vi "浊度电极校准.vi"() -> ()   [LabVIEW 2016, in "斯坦道多参数.lvlib"]
uses:
  <vilib>/Utility/miscctls.llb/LVPointTypeDef.ctl
  <vilib>/Utility/miscctls.llb/LVPositionTypeDef.ctl
  <vilib>/Analysis/NI_AALBase.lvlib
panel:
  out "通讯状态":string
  out "电极状态标志":u16(ring) items=["OK"=0, "第一点校正通过"=1, "第二点校正通过"=2, "悬浮物两点校准第一点校正通过"=11, "悬浮物两点校准第二点校正通过"=12, "浊度三点校正第一点校正通过"=31, "浊度三点校正第二点校正通过"=32, "浊度三点校正第三点校正通过"=33]
  out "第三点校准值":dbl
  out "标液3":dbl
  out "第二点校准值":dbl
  out "第一点校准值":dbl
  in  "校准停止":bool
  in  "校准启动":bool
  in  "校准模式":enum16{"两点校准", "单点校准", "三点校准"}(ring)
  out "最小值":sgl format="%#.2f"
  out "最大值":sgl format="%#.2f"
  out "波形图表":sgl(graph) caption="历史曲线"
  out "mean":dbl caption="均值" format="%#.2f"
  out "standard deviation":dbl caption="标准差" format="%#.2f"
  out "变异系数":dbl format="%#.6f"
  out "测量值":dbl
  out "提示":string
  out "标液2":dbl
  out "标液1":dbl
  out "原始读取值":dbl caption="信号值"
  out "偏移值补偿":dbl
  out "电极斜率":dbl
  out "电极零点":dbl
  # "浊度电极设定"
  # "NTU"
  # "%"
  # "NTU"
  # "NTU"
  # "NTU"
  # "请选择校准模式:"
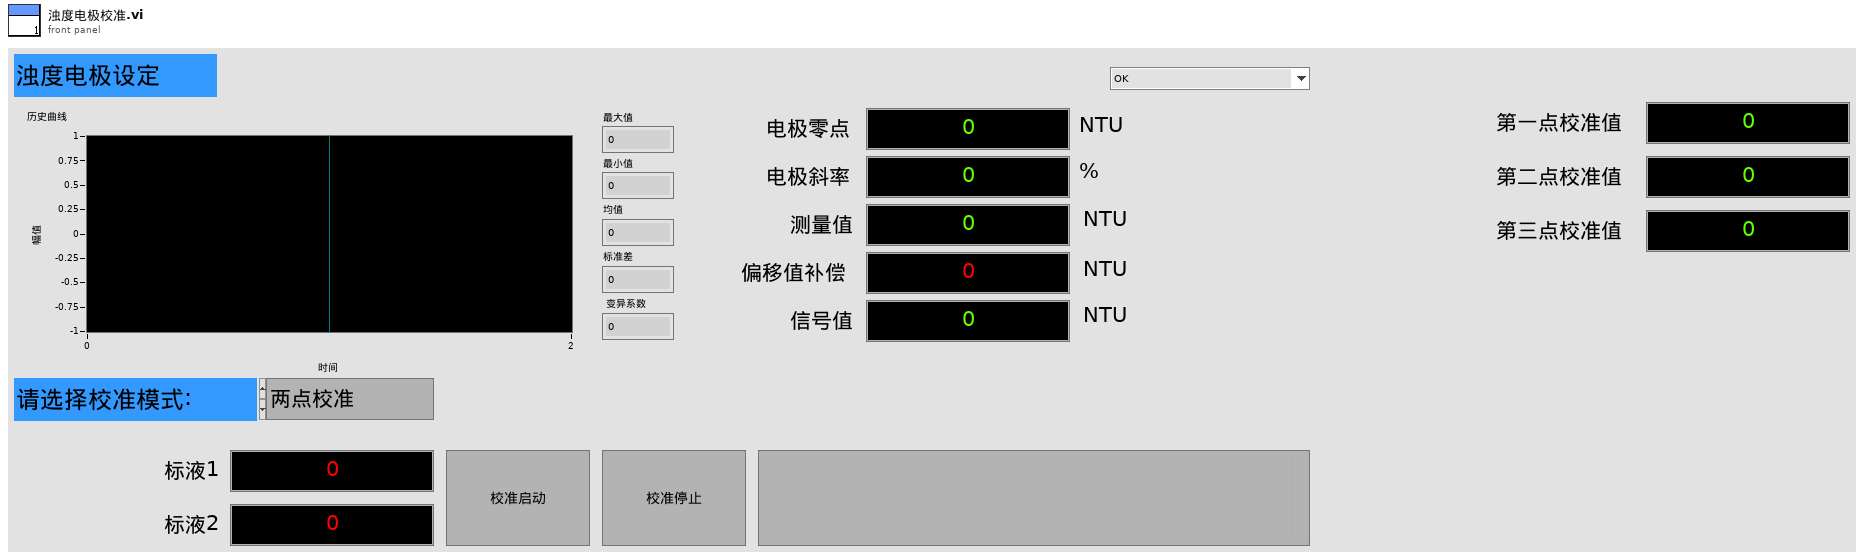
[diagram p1: front panel]
types:
  T1 = typedef "LVPointTypeDef.ctl" = cluster{"Horizontal":i16, "Vertical":i16}
  T2 = typedef "斯坦道多参数.lvlib/校准步骤.ctl" = enum16{"待机", "放置第一点标液", "第一点校准启动", "第一点校准写入", "第一点校准失败", "放置第二点标液", "第二点校准启动", "第二点校准写入", "第二点校准失败", "放置第三点标液", "第三点校准启动", "第三点校准写入", "第三点校准失败", "校准结果写入", "校准结束"}
  T3 = cluster{"电极状态标志":u16, "电极型号标志":u16, "浊度测量值":sgl, "温度测量值":sgl, "浊度信号值":sgl, "浊度偏移修正值":sgl, "温度偏移修正值":sgl, "手动温度补偿值":sgl, "浊度电极零点":sgl, "浊度电极斜率":sgl, "第1点标准值记录":sgl, "第1点信号值记录":sgl, "第1点温度值记录":sgl, "第2点标准值记录":sgl, "第2点信号值记录":sgl, "第2点温度值记录":sgl, "命令滤波设定":u16, "温度模式":enum16{"ATC", "MTC"}, "生产批次":u16, "电极序号":u16, "串口地址":u16, "串口波特率":enum16{"9600", "19200", "115200"}, "串口校验位":enum16{"NONE", "ODD", "EVEN"}, "串口停止位":enum16{"1bit", "2bit"}, "第一点标准值":sgl, "第二点标准值":sgl, "第三点标准值":sgl}
  T4 = typedef "LVPositionTypeDef.ctl" = cluster{"Left":i32, "Top":i32}
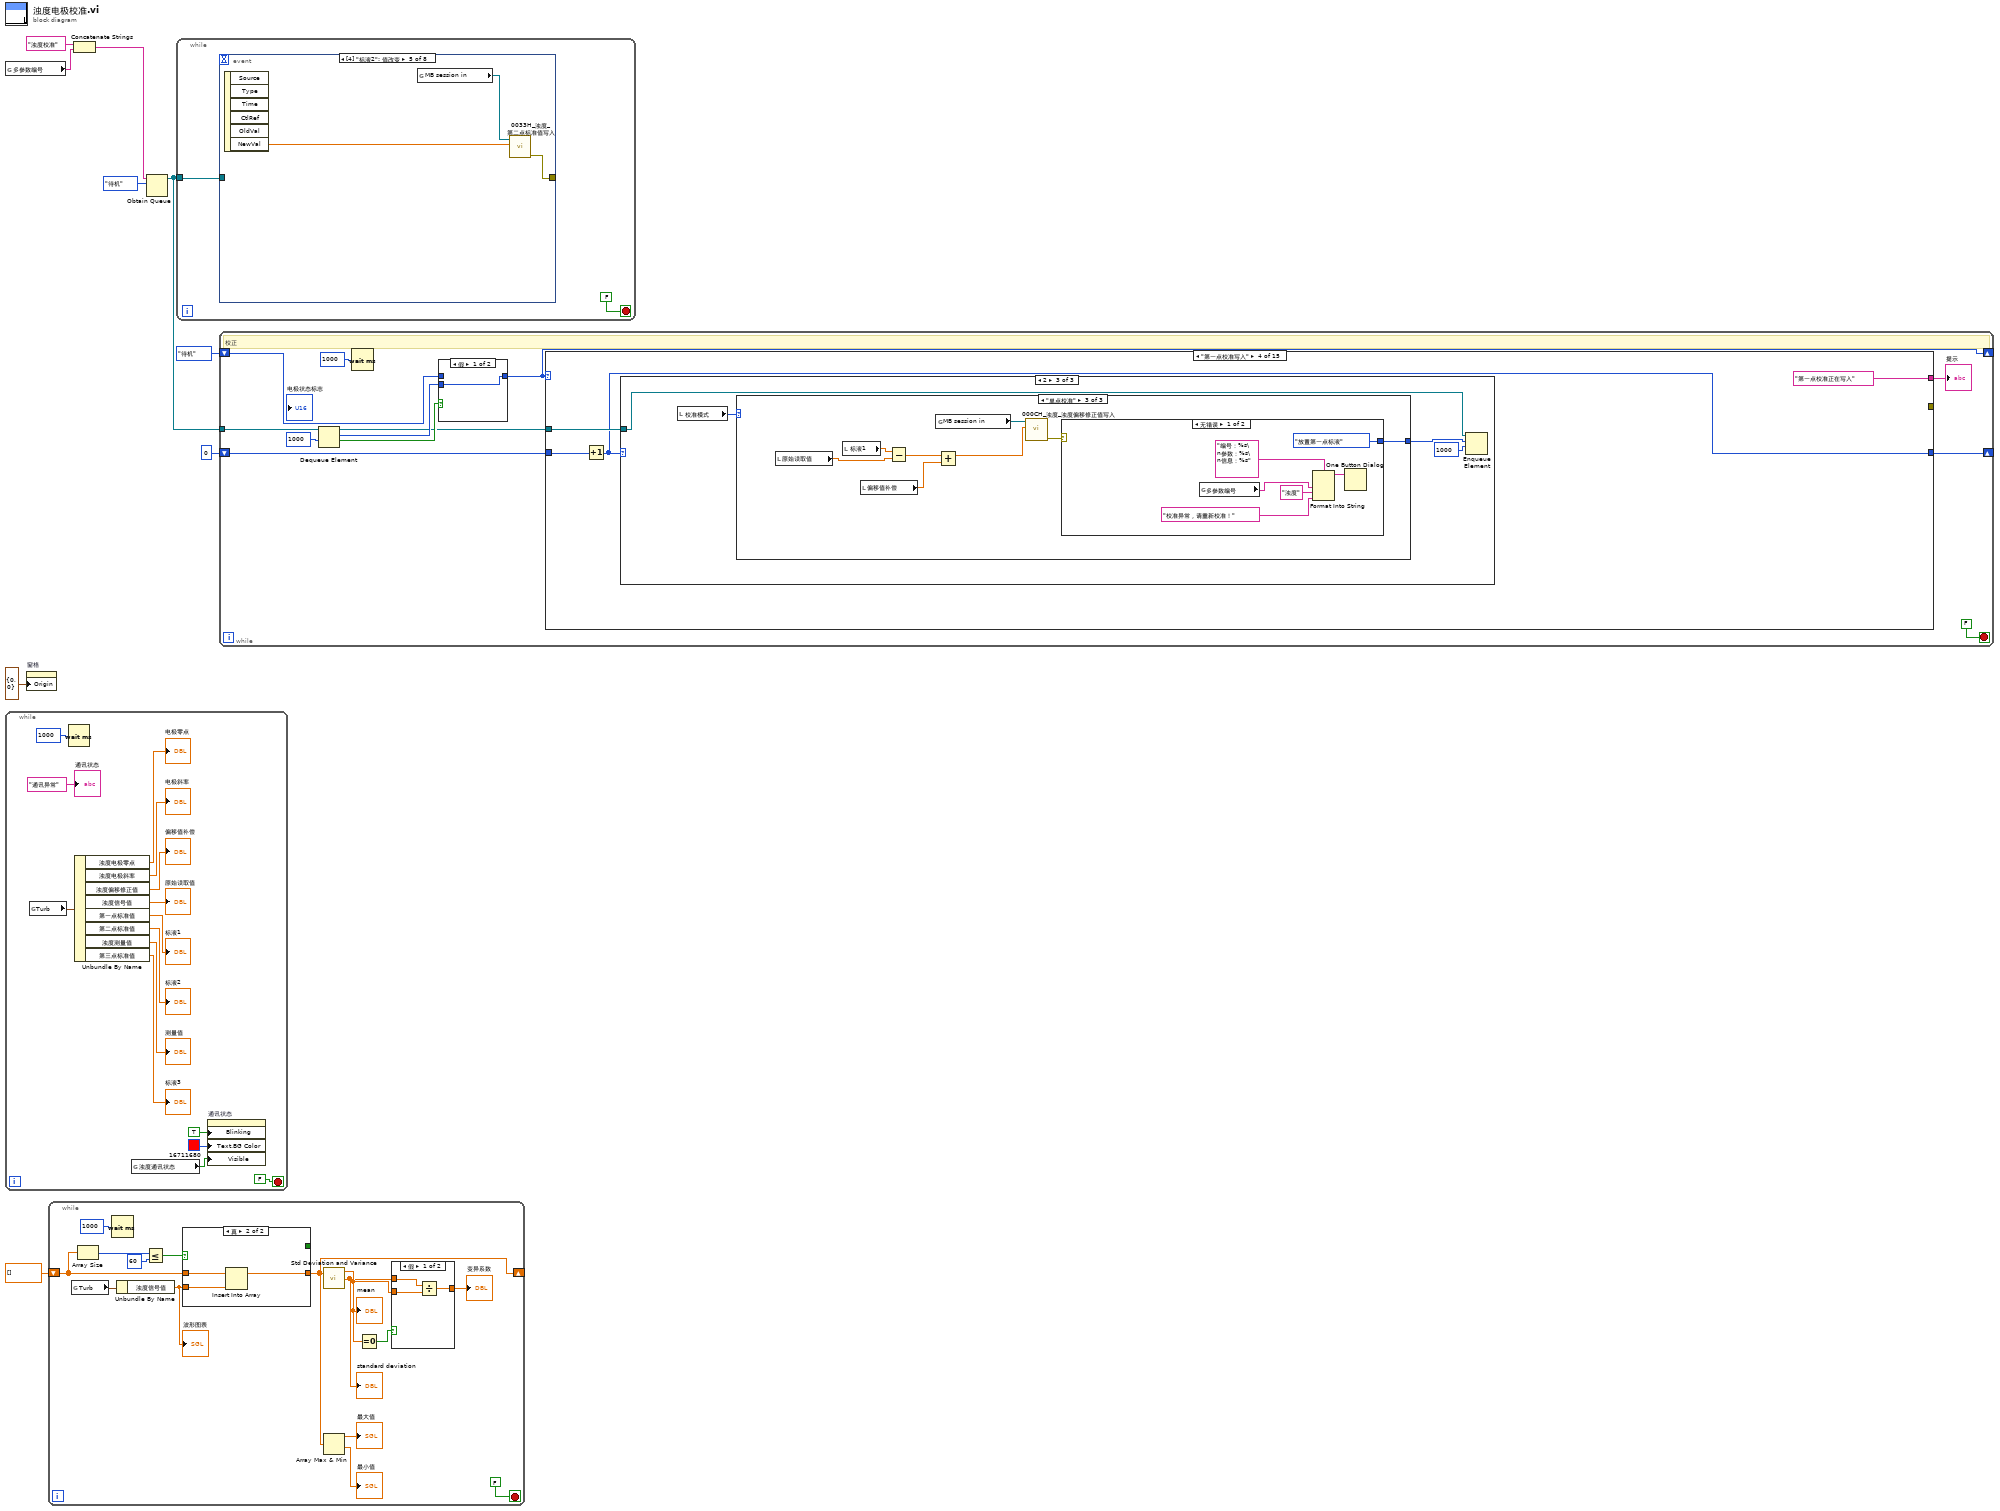
[diagram p0: block diagram]
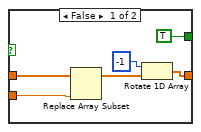
[diagram p3: hidden frame]
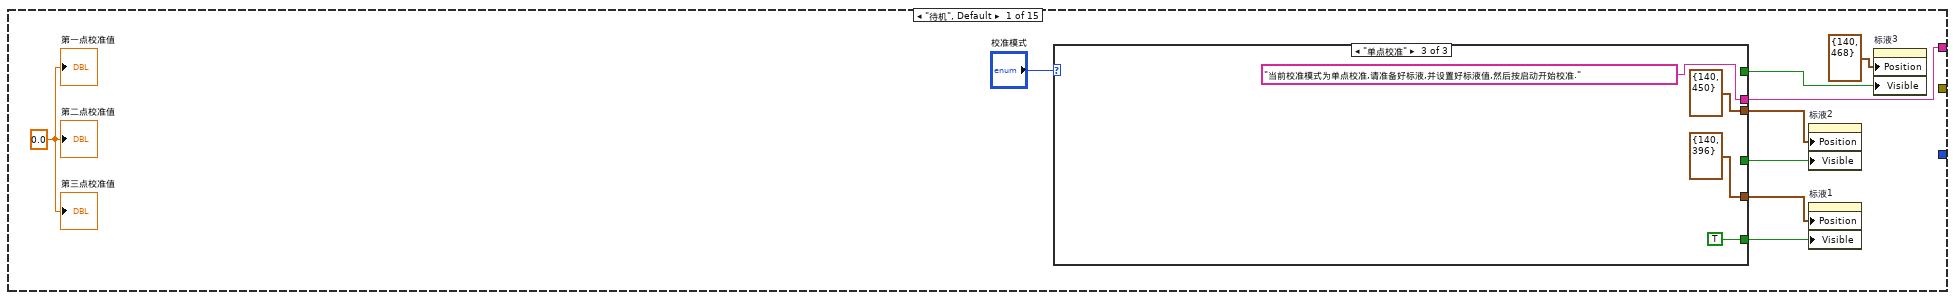
[diagram p5: hidden frame]
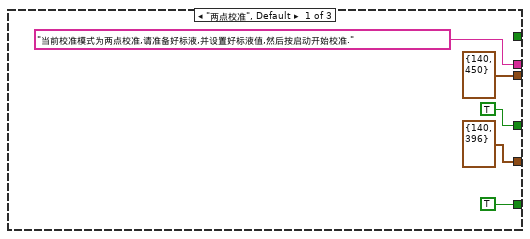
[diagram p6: hidden frame]
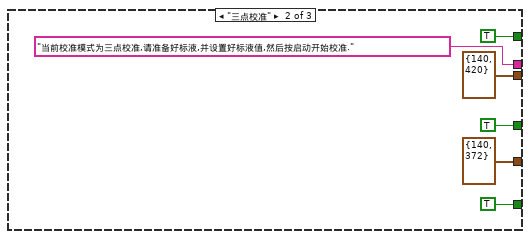
[diagram p7: hidden frame]
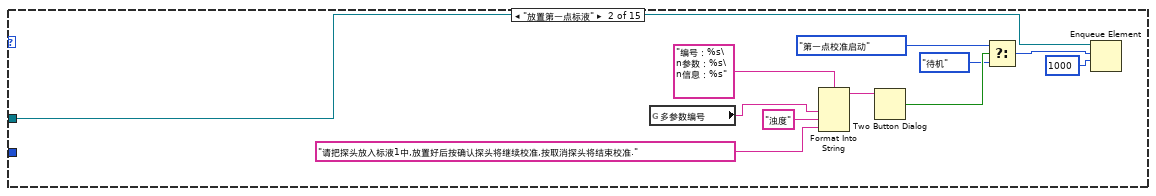
[diagram p8: hidden frame]
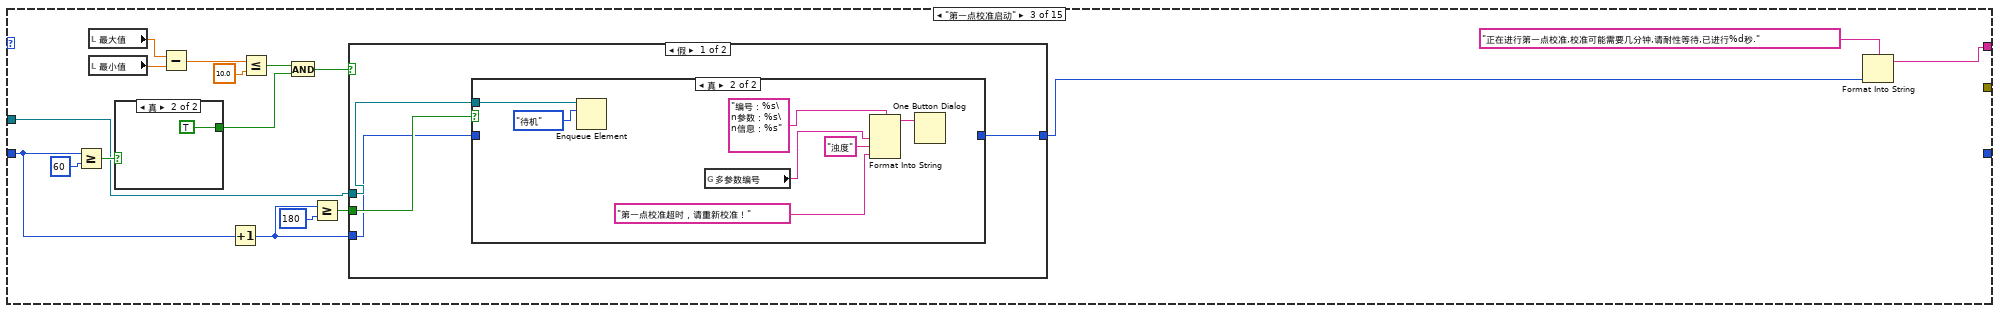
[diagram p9: hidden frame]
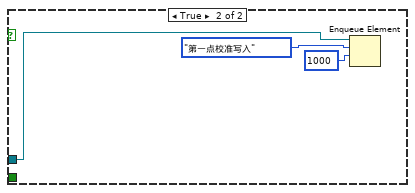
[diagram p11: hidden frame]
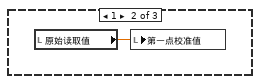
[diagram p14: hidden frame]
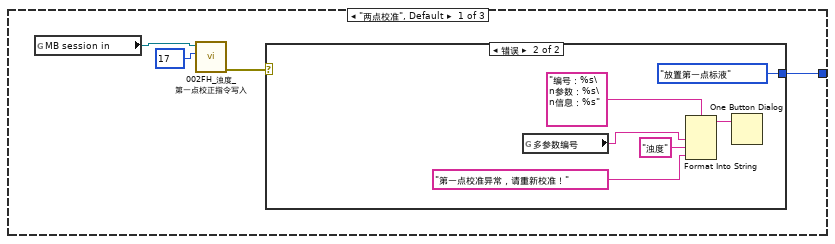
[diagram p15: hidden frame]
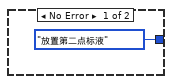
[diagram p16: hidden frame]
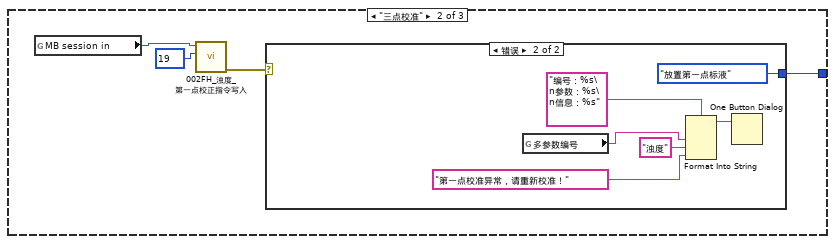
[diagram p17: hidden frame]
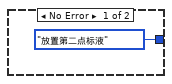
[diagram p18: hidden frame]
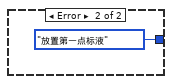
[diagram p19: hidden frame]
diagram:
  n1 = global read "多参数全局变量.vi" "多参数编号"() -> (w1:string)
  n2 = while {
    stop <- FALSE stop-if-true
    n3 = global read "国弘过程全局变量.vi" "Turb"() -> (w22:T3)
    n4 = Wait (ms)(milliseconds to wait=u32 1000 ("等待时间（毫秒）")) -> ()  [unwired: 1 out]
    n5 = Unbundle By Name(w22) -> ("浊度电极零点"=→"电极零点":sgl, "浊度电极斜率"=→"电极斜率":sgl, "浊度偏移修正值"=→"偏移值补偿":sgl, "浊度信号值"=→"原始读取值":sgl, "第一点标准值"=→"标液1":sgl, "第二点标准值"=→"标液2":sgl, "浊度测量值"=→"测量值":sgl, "第三点标准值"=→"标液3":sgl)
    n6 = global read "多参数全局变量.vi" "浊度通讯状态"() -> (w10:bool)
    n7 = property on="通讯状态" class="Str"("Blinking"=TRUE ("闪烁"), "Text.BG Color"=u32 16711680, "Visible"=w10) -> ()  [unwired: 2 in, 2 out]
    "通讯状态" <- "通讯异常" ("当前串口")
  }
  n8 = property on="窗格" class="Pane"("Origin"=T1 {"Horizontal"=0, "Vertical"=0} ("原点")) -> ()  [unwired: 2 in, 2 out]
  n9 = while {
    shift-right: [w28] -> _
    shift-left: sgl[] [] -> [w35]
    stop <- FALSE stop-if-true
    n10 = global read "国弘过程全局变量.vi" "Turb"() -> (w29:T3)
    n11 = Array Size(array=w35) -> (size(s)=w37:i32)
    n12 = Wait (ms)(milliseconds to wait=u32 1000 ("等待时间（毫秒）")) -> ()  [unwired: 1 out]
    n13 = Unbundle By Name(w29) -> ("浊度信号值"=w25:sgl)
    "波形图表" <- w25
    n14 = Less Or Equal?(x=w37, y=60) -> (x <= y?=w36:bool)
    n15 = case shown="真" w36 {
      tunnel: w35 -> [w48 w51]
      tunnel: w25 -> [w46 w50]
      tunnel: [w44 w49] -> w28
      tunnel: [TRUE _] -> _
      frame False {
        n16 = Replace Array Subset(array=w48, new element=w46) -> (w47:sgl[])  [unwired: 1 in]
        n17 = Rotate 1D Array(1:w47, 2:-1 ("n")) -> (0:w44:sgl[])
      }
      frame True {
        n18 = Insert Into Array(array=w51, new element=w50) -> (w49:sgl[])  [unwired: 1 in]
      }
    }
    n19 = call <vilib>:"Std Deviation and Variance.vi"("X"=w28) -> ("mean"=w33:dbl, "standard deviation"=w32:dbl)  [unwired: 1 in, 1 out]
    "mean" <- w33
    "standard deviation" <- w32
    n20 = Array Max & Min(array=w28) -> (max value=→"最大值":sgl, min value=→"最小值":sgl)  [unwired: 2 out]
    n21 = Equal To 0?(x=w33) -> (x = 0?=w34:bool)
    n22 = case shown="假" w34 {
      tunnel: w32 -> [w42 _]
      tunnel: [w41 _] -> w31
      tunnel: w33 -> [w40 _]
      frame False {
        n23 = Divide(x=w42, y=w40) -> (x/y=w41:dbl)
      }
      frame True {
      }
    }
    "变异系数" <- w31
  }
  n24 = Concatenate Strings("浊度校准" ("名称（未命名）"), w1) -> (w2:string)
  n25 = Obtain Queue(name (unnamed)=w2, element data type=校准步骤."待机" ("枚举")) -> (queue out=w4:refnum<queue>)  [unwired: 3 in, 2 out]
  n26 = while {
    tunnel: w4 -> [w52]
    stop <- FALSE stop-if-true
    n27 = event shown="[4] \"标液2\": 值改变" {
      selector: _ -> [_ _ _ _ _ _ _ _]
      dyn-events: _ -> [_ _ _ _ _ _ _ _]
      timeout: _ -> [_ _ _ _ _ _ _ _]
      tunnel: [_ _ w59 w62 w66 w69 _ _] -> _
      tunnel: w52 -> [_ _ _ _ _ _ w70 w72]
      event Timeout {
        n28 = event-data() -> ()  [unwired: 1 in, 3 out]
      }
      event "偏移值补偿", "标液1", "标液2", "标液3": Mouse Down {
        n29 = event-data() -> ("CtlRef"=w54:refnum<vi>)  [unwired: 1 in, 7 out]
        n30 = property class="DigNum (严格)"(reference=w54) -> (reference out=w55:refnum<vi>, "Value"=w56:dbl)  [unwired: 1 in, 1 out]
        n31 = call "数字键盘.vi"("OldNumber"=w56) -> ("NewNumber"=w57:dbl)  [unwired: 1 in]
        n32 = property class="DigNum (严格)"(reference=w55, "Val(Sgnl)"=w57) -> ()  [unwired: 1 in, 2 out]
      }
      event "偏移值补偿": Value Change {
        n33 = event-data() -> ("NewVal"=w60:dbl)  [unwired: 1 in, 5 out]
        n34 = global read "多参数全局变量.vi" "MB session in"() -> (w58:refnum<class "MB_Master.lvclass">)
        n35 = call "000CH_浊度_浊度偏移修正值写入.vi"("数值"=w60, "MB session in"=w58) -> ("error out"=w59:errorcluster)  [unwired: 8 in, 1 out]
      }
      event "标液1": Value Change {
        n36 = event-data() -> ("NewVal"=w63:dbl)  [unwired: 1 in, 5 out]
        n37 = global read "多参数全局变量.vi" "MB session in"() -> (w61:refnum<class "MB_Master.lvclass">)
        n38 = call "0030H_浊度_第一点标准值写入.vi"("数值"=w63, "MB session in"=w61) -> ("error out"=w62:errorcluster)  [unwired: 8 in, 1 out]
      }
      event "标液2": Value Change {
        n39 = event-data() -> ("NewVal"=w65:dbl)  [unwired: 1 in, 5 out]
        n40 = global read "多参数全局变量.vi" "MB session in"() -> (w64:refnum<class "MB_Master.lvclass">)
        n41 = call "0033H_浊度_第二点标准值写入.vi"("数值"=w65, "MB session in"=w64) -> ("error out"=w66:errorcluster)  [unwired: 8 in, 1 out]
      }
      event "标液3": Value Change {
        n42 = event-data() -> ("NewVal"=w68:dbl)  [unwired: 1 in, 5 out]
        n43 = global read "多参数全局变量.vi" "MB session in"() -> (w67:refnum<class "MB_Master.lvclass">)
        n44 = call "0036H_浊度_第三点标准值写入.vi"("数值"=w68, "MB session in"=w67) -> ("error out"=w69:errorcluster)  [unwired: 8 in, 1 out]
      }
      event "校准启动": Value Change {
        n45 = event-data() -> ()  [unwired: 1 in, 6 out]
        n46 = Enqueue Element(queue=w70, element=校准步骤."放置第一点标液" ("元素")) -> ()  [unwired: 2 in, 3 out]
      }
      event "校准停止": Value Change {
        n47 = event-data() -> ()  [unwired: 1 in, 6 out]
        n48 = Flush Queue(queue=w72) -> (queue out=w73:refnum<queue>)  [unwired: 1 in, 2 out]
        n49 = Enqueue Element(queue=w73, element=校准步骤."待机" ("元素"), timeout in ms (-1)=1000 ("超时毫秒(-1)")) -> ()  [unwired: 1 in, 3 out]
      }
    }
  }
  n50 = while "While循环" {
    shift-right: [w77] -> _
    shift-left: 校准步骤."待机" ("枚举") -> [w79]
    shift-right: [w76] -> _
    shift-left: 0 -> [w85]
    tunnel: w4 -> [w80]
    stop <- FALSE stop-if-true
    # "校正"
    n51 = Dequeue Element(queue=w80, timeout in ms (-1)=1000 ("超时毫秒(-1)")) -> (queue out=w78:refnum<queue>, element=w81:T2, timed out?=w82:bool)  [unwired: 1 in, 1 out]
    n52 = Wait (ms)(milliseconds to wait=u32 1000 ("等待时间（毫秒）")) -> ()  [unwired: 1 out]
    n53 = case shown="假" w82 {
      tunnel: w81 -> [w88 _]
      tunnel: [w88 w89] -> w77
      tunnel: w79 -> [_ w89]
      frame False {
      }
      frame True {
      }
    }
    n54 = case shown="\"第一点校准写入\"" w77 {
      tunnel: [w97 _ w125 "第一点校准正在写入" ("提示") _ _ w217 "第二点校准正在写入" ("提示") "第二点校准失败" ("提示") _ "第三点校准正在写入" ("提示") w313 "第三点校准失败" ("提示") w347 w386] -> w84
      tunnel: w85 -> [_ _ w127 w160 _ _ w218 w250 _ _ w295 w314 _ _ _]
      tunnel: [_ _ _ w158 _ _ w216 w248 _ _ w293 w312 _ _ _] -> w76
      tunnel: w78 -> [_ w119 w128 w159 _ w209 w219 w249 _ w287 w294 w315 _ w354 _]
      tunnel: [_ _ _ _ _ _ _ _ _ _ _ _ _ w352 _] -> _
      frame "待机", Default {
        w90 = 0.0 ("第一点校准值")
        n55 = case shown="\"单点校准\"" "校准模式" {
          tunnel: ["当前校准模式为两点校准,请准备好标液,并设置好标液值,然后按启动开始校准." ("提示") "当前校准模式为三点校准,请准备好标液,并设置好标液值,然后按启动开始校准." ("提示") "当前校准模式为单点校准,请准备好标液,并设置好标液值,然后按启动开始校准." ("提示")] -> w97
          tunnel: [TRUE ("可见") TRUE ("可见") _] -> w93
          tunnel: [T4 {"Left"=140, "Top"=396} ("位置") T4 {"Left"=140, "Top"=372} ("位置") T4 {"Left"=140, "Top"=396} ("位置")] -> w96
          tunnel: [T4 {"Left"=140, "Top"=450} ("位置 2") T4 {"Left"=140, "Top"=420} ("位置 2") T4 {"Left"=140, "Top"=450} ("位置 2")] -> w95
          tunnel: [_ TRUE ("可见") _] -> w92
          tunnel: [TRUE ("可见") TRUE ("可见") TRUE ("可见")] -> w91
          frame "两点校准", Default {
          }
          frame "三点校准" {
          }
          frame "单点校准" {
          }
        }
        n56 = property on="标液2" class="DigNum (严格)"("Position"=w95, "Visible"=w93) -> ()  [unwired: 2 in, 2 out]
        n57 = property on="标液1" class="DigNum (严格)"("Position"=w96, "Visible"=w91) -> ()  [unwired: 2 in, 2 out]
        n58 = property on="标液3" class="DigNum (严格)"("Position"=T4 {"Left"=140, "Top"=468} ("位置 3"), "Visible"=w92) -> ()  [unwired: 2 in, 2 out]
        "第一点校准值" <- w90
        "第二点校准值" <- w90
        "第三点校准值" <- w90
      }
      frame "放置第一点标液" {
        n59 = global read "多参数全局变量.vi" "多参数编号"() -> (w117:string)
        n60 = Format Into String(format string="编号：%s\n参数：%s\n信息：%s" ("格式字符串"), w117, "浊度" ("输入 2"), "请把探头放入标液1中,放置好后按确认探头将继续校准,按取消探头将结束校准." ("消息")) -> (resulting string=w114:string)  [unwired: 2 in, 1 out]
        n61 = Two Button Dialog(message=w114) -> (T button?=w123:bool)  [unwired: 2 in]
        n62 = Select(t=校准步骤."第一点校准启动" ("元素"), s=w123, f=校准步骤."待机" ("元素")) -> (s? t:f=w120:T2)
        n63 = Enqueue Element(queue=w119, element=w120, timeout in ms (-1)=1000 ("超时毫秒(-1)")) -> ()  [unwired: 1 in, 3 out]
      }
      frame "第一点校准启动" {
        n64 = Greater Or Equal?(x=w127, y=60) -> (x >= y?=w134:bool)
        n65 = local read "最大值"() -> (w137:sgl)
        n66 = local read "最小值"() -> (w136:sgl)
        n67 = case shown="真" w134 {
          tunnel: [_ TRUE] -> w135
          frame False {
          }
          frame True {
          }
        }
        n68 = Subtract(x=w137, y=w136) -> (x-y=w138:sgl)
        n69 = Increment(x=w127) -> (x+1=w141:i32)
        n70 = Less Or Equal?(x=w138, y=10.0) -> (x <= y?=w131:bool)
        n71 = And(x=w131, y=w135) -> (x .and. y?=w139:bool)
        n72 = Greater Or Equal?(x=w141, y=180) -> (x >= y?=w140:bool)
        n73 = case shown="假" w139 {
          tunnel: w128 -> [w144 w156]
          tunnel: w140 -> [w145 _]
          tunnel: w141 -> [w143 _]
          tunnel: [w142 _] -> w126
          frame False {
            n74 = case shown="真" w145 {
              tunnel: w144 -> [_ w153]
              tunnel: w143 -> [w146 _]
              tunnel: [w146 _] -> w142
              frame False {
              }
              frame True {
                n75 = Enqueue Element(queue=w153, element=校准步骤."待机" ("元素")) -> ()  [unwired: 2 in, 3 out]
                n76 = global read "多参数全局变量.vi" "多参数编号"() -> (w150:string)
                n77 = Format Into String(format string="编号：%s\n参数：%s\n信息：%s" ("格式字符串"), w150, "浊度" ("输入 2"), "第一点校准超时，请重新校准！" ("error source (\" \")")) -> (resulting string=w148:string)  [unwired: 2 in, 1 out]
                n78 = One Button Dialog(message=w148) -> ()  [unwired: 1 in, 1 out]
              }
            }
          }
          frame True {
            n79 = Enqueue Element(queue=w156, element=校准步骤."第一点校准写入" ("元素"), timeout in ms (-1)=1000 ("超时毫秒(-1)")) -> ()  [unwired: 1 in, 3 out]
          }
        }
        n80 = Format Into String(format string="正在进行第一点校准,校准可能需要几分钟,请耐性等待,已进行%d秒." ("格式字符串"), w126) -> (resulting string=w125:string)  [unwired: 2 in, 1 out]
      }
      frame "第一点校准写入" {
        n81 = Increment(x=w160) -> (x+1=w158:i32)
        n82 = case shown="2" w158 {
          tunnel: w159 -> [_ _ w166]
          frame 0, Default {
          }
          frame 1 {
            n83 = local read "原始读取值"() -> (w162:dbl)
            n84 = local write "第一点校准值"(w162) -> ()
          }
          frame 2 {
            n85 = local read "校准模式"() -> (w165:enum16{"两点校准", "单点校准", "三点校准"})
            n86 = case shown="\"单点校准\"" w165 {
              tunnel: [w167 w178 w191] -> w164
              frame "两点校准", Default {
                n87 = global read "多参数全局变量.vi" "MB session in"() -> (w170:refnum<class "MB_Master.lvclass">)
                n88 = call "002FH_浊度_第一点校正指令写入.vi"("数值"=u16 17, "MB session in"=w170) -> ("error out"=w168:errorcluster)  [unwired: 8 in, 1 out]
                n89 = case shown="错误" w168 {
                  tunnel: [校准步骤."放置第二点标液" ("元素") 校准步骤."放置第一点标液" ("元素")] -> w167
                  frame No Error {
                  }
                  frame Error {
                    n90 = global read "多参数全局变量.vi" "多参数编号"() -> (w176:string)
                    n91 = Format Into String(format string="编号：%s\n参数：%s\n信息：%s" ("格式字符串"), w176, "浊度" ("输入 2"), "第一点校准异常，请重新校准！" ("error source (\" \")")) -> (resulting string=w175:string)  [unwired: 2 in, 1 out]
                    n92 = One Button Dialog(message=w175) -> ()  [unwired: 1 in, 1 out]
                  }
                }
              }
              frame "三点校准" {
                n93 = global read "多参数全局变量.vi" "MB session in"() -> (w181:refnum<class "MB_Master.lvclass">)
                n94 = call "002FH_浊度_第一点校正指令写入.vi"("数值"=u16 19, "MB session in"=w181) -> ("error out"=w179:errorcluster)  [unwired: 8 in, 1 out]
                n95 = case shown="错误" w179 {
                  tunnel: [校准步骤."放置第二点标液" ("元素") 校准步骤."放置第一点标液" ("元素")] -> w178
                  frame No Error {
                  }
                  frame Error {
                    n96 = global read "多参数全局变量.vi" "多参数编号"() -> (w187:string)
                    n97 = Format Into String(format string="编号：%s\n参数：%s\n信息：%s" ("格式字符串"), w187, "浊度" ("输入 2"), "第一点校准异常，请重新校准！" ("error source (\" \")")) -> (resulting string=w186:string)  [unwired: 2 in, 1 out]
                    n98 = One Button Dialog(message=w186) -> ()  [unwired: 1 in, 1 out]
                  }
                }
              }
              frame "单点校准" {
                n99 = local read "原始读取值"() -> (w196:dbl)
                n100 = local read "标液1"() -> (w195:dbl)
                n101 = local read "偏移值补偿"() -> (w189:dbl)
                n102 = Subtract(x=w195, y=w196) -> (x-y=w193:dbl)
                n103 = global read "多参数全局变量.vi" "MB session in"() -> (w194:refnum<class "MB_Master.lvclass">)
                n104 = Add(x=w193, y=w189) -> (x+y=w190:dbl)
                n105 = call "000CH_浊度_浊度偏移修正值写入.vi"("数值"=w190, "MB session in"=w194) -> ("error out"=w192:errorcluster)  [unwired: 8 in, 1 out]
                n106 = case shown="无错误" w192 {
                  tunnel: [校准步骤."放置第一点标液" ("元素") 校准步骤."放置第一点标液" ("元素")] -> w191
                  frame No Error {
                    n107 = global read "多参数全局变量.vi" "多参数编号"() -> (w199:string)
                    n108 = Format Into String(format string="编号：%s\n参数：%s\n信息：%s" ("格式字符串"), w199, "浊度" ("输入 2"), "校准异常，请重新校准！" ("error source (\" \")")) -> (resulting string=w200:string)  [unwired: 2 in, 1 out]
                    n109 = One Button Dialog(message=w200) -> ()  [unwired: 1 in, 1 out]
                  }
                  frame Error {
                  }
                }
              }
            }
            n110 = Enqueue Element(queue=w166, element=w164, timeout in ms (-1)=1000 ("超时毫秒(-1)")) -> ()  [unwired: 1 in, 3 out]
          }
        }
      }
      frame "第一点校准失败" {
      }
      frame "放置第二点标液" {
        n111 = global read "多参数全局变量.vi" "多参数编号"() -> (w207:string)
        n112 = Format Into String(format string="编号：%s\n参数：%s\n信息：%s" ("格式字符串"), w207, "浊度" ("输入 2"), "请把探头放入标液2中,放置好后按确认探头将继续校准,按取消探头将结束校准." ("消息")) -> (resulting string=w204:string)  [unwired: 2 in, 1 out]
        n113 = Two Button Dialog(message=w204) -> (T button?=w213:bool)  [unwired: 2 in]
        n114 = Select(t=校准步骤."第二点校准启动" ("元素"), s=w213, f=校准步骤."待机" ("元素")) -> (s? t:f=w210:T2)
        n115 = Enqueue Element(queue=w209, element=w210, timeout in ms (-1)=1000 ("超时毫秒(-1)")) -> ()  [unwired: 1 in, 3 out]
      }
      frame "第二点校准启动" {
        n116 = Greater Or Equal?(x=w218, y=60) -> (x >= y?=w224:bool)
        n117 = local read "最大值"() -> (w227:sgl)
        n118 = local read "最小值"() -> (w226:sgl)
        n119 = case shown="真" w224 {
          tunnel: [_ TRUE] -> w225
          frame False {
          }
          frame True {
          }
        }
        n120 = Subtract(x=w227, y=w226) -> (x-y=w228:sgl)
        n121 = Increment(x=w218) -> (x+1=w231:i32)
        n122 = Less Or Equal?(x=w228, y=10.0) -> (x <= y?=w221:bool)
        n123 = And(x=w221, y=w225) -> (x .and. y?=w229:bool)
        n124 = Greater Or Equal?(x=w231, y=180) -> (x >= y?=w230:bool)
        n125 = case shown="假" w229 {
          tunnel: w219 -> [w234 w246]
          tunnel: w230 -> [w235 _]
          tunnel: w231 -> [w233 _]
          tunnel: [w232 _] -> w216
          frame False {
            n126 = case shown="真" w235 {
              tunnel: w234 -> [_ w243]
              tunnel: w233 -> [w236 _]
              tunnel: [w236 _] -> w232
              frame False {
              }
              frame True {
                n127 = Enqueue Element(queue=w243, element=校准步骤."放置第二点标液" ("元素")) -> ()  [unwired: 2 in, 3 out]
                n128 = global read "多参数全局变量.vi" "多参数编号"() -> (w240:string)
                n129 = Format Into String(format string="编号：%s\n参数：%s\n信息：%s" ("格式字符串"), w240, "浊度" ("输入 2"), "第二点校准超时，请重新校准！" ("error source (\" \")")) -> (resulting string=w238:string)  [unwired: 2 in, 1 out]
                n130 = One Button Dialog(message=w238) -> ()  [unwired: 1 in, 1 out]
              }
            }
          }
          frame True {
            n131 = Enqueue Element(queue=w246, element=校准步骤."第二点校准写入" ("元素"), timeout in ms (-1)=1000 ("超时毫秒(-1)")) -> ()  [unwired: 1 in, 3 out]
          }
        }
        n132 = Format Into String(format string="正在进行第二点校准,校准可能需要几分钟,请耐性等待,已进行%d秒." ("格式字符串"), w216) -> (resulting string=w217:string)  [unwired: 2 in, 1 out]
      }
      frame "第二点校准写入" {
        n133 = Increment(x=w250) -> (x+1=w248:i32)
        n134 = case shown="0, 默认" w248 {
          tunnel: w249 -> [_ _ w256]
          frame 0, Default {
          }
          frame 1 {
            n135 = local read "原始读取值"() -> (w252:dbl)
            n136 = local write "第二点校准值"(w252) -> ()
          }
          frame 2 {
            n137 = local read "校准模式"() -> (w253:enum16{"两点校准", "单点校准", "三点校准"})
            n138 = case shown="\"三点校准\"" w253 {
              tunnel: [w260 w271] -> w254
              frame "两点校准", Default {
                n139 = global read "多参数全局变量.vi" "MB session in"() -> (w257:refnum<class "MB_Master.lvclass">)
                n140 = call "0032H_浊度_第二点校正指令写入.vi"("数值"=u16 33, "MB session in"=w257) -> ("error out"=w258:errorcluster)  [unwired: 8 in, 1 out]
                n141 = case shown="错误" w258 {
                  tunnel: [校准步骤."校准结果写入" ("元素") 校准步骤."放置第二点标液" ("元素")] -> w260
                  frame No Error {
                  }
                  frame Error {
                    n142 = global read "多参数全局变量.vi" "多参数编号"() -> (w265:string)
                    n143 = Format Into String(format string="编号：%s\n参数：%s\n信息：%s" ("格式字符串"), w265, "浊度" ("输入 2"), "第二点校准异常，请重新校准！" ("error source (\" \")")) -> (resulting string=w264:string)  [unwired: 2 in, 1 out]
                    n144 = One Button Dialog(message=w264) -> ()  [unwired: 1 in, 1 out]
                  }
                }
              }
              frame "三点校准" {
                n145 = global read "多参数全局变量.vi" "MB session in"() -> (w268:refnum<class "MB_Master.lvclass">)
                n146 = call "0032H_浊度_第二点校正指令写入.vi"("数值"=u16 35, "MB session in"=w268) -> ("error out"=w269:errorcluster)  [unwired: 8 in, 1 out]
                n147 = case shown="错误" w269 {
                  tunnel: [校准步骤."放置第三点标液" ("元素") 校准步骤."放置第二点标液" ("元素")] -> w271
                  frame No Error {
                  }
                  frame Error {
                    n148 = global read "多参数全局变量.vi" "多参数编号"() -> (w276:string)
                    n149 = Format Into String(format string="编号：%s\n参数：%s\n信息：%s" ("格式字符串"), w276, "浊度" ("输入 2"), "第二点校准异常，请重新校准！" ("error source (\" \")")) -> (resulting string=w275:string)  [unwired: 2 in, 1 out]
                    n150 = One Button Dialog(message=w275) -> ()  [unwired: 1 in, 1 out]
                  }
                }
              }
            }
            n151 = Enqueue Element(queue=w256, element=w254, timeout in ms (-1)=1000 ("超时毫秒(-1)")) -> ()  [unwired: 1 in, 3 out]
          }
        }
      }
      frame "第二点校准失败" {
      }
      frame "放置第三点标液" {
        n152 = global read "多参数全局变量.vi" "多参数编号"() -> (w283:string)
        n153 = global read "多参数全局变量.vi" "多参数编号"() -> (w285:string)
        n154 = Format Into String(format string="编号：%s\n参数：%s\n信息：%s" ("格式字符串"), w283, "浊度" ("输入 2"), "请把探头放入标液3中,放置好后按确认探头将继续校准,按取消探头将结束校准." ("消息")) -> (resulting string=w280:string)  [unwired: 2 in, 1 out]
        n155 = Concatenate Strings(w285, w280) -> (w286:string)
        n156 = Two Button Dialog(message=w286) -> (T button?=w291:bool)  [unwired: 2 in]
        n157 = Select(t=校准步骤."第三点校准启动" ("元素"), s=w291, f=校准步骤."待机" ("元素")) -> (s? t:f=w288:T2)
        n158 = Enqueue Element(queue=w287, element=w288, timeout in ms (-1)=1000 ("超时毫秒(-1)")) -> ()  [unwired: 1 in, 3 out]
      }
      frame "第三点校准写入" {
        n159 = Increment(x=w295) -> (x+1=w293:i32)
        n160 = case shown="1" w293 {
          tunnel: w294 -> [_ _ w303]
          frame 0, Default {
          }
          frame 1 {
            n161 = local read "原始读取值"() -> (w297:dbl)
            n162 = local write "第二点校准值"(w297) -> ()
          }
          frame 2 {
            n163 = global read "多参数全局变量.vi" "MB session in"() -> (w298:refnum<class "MB_Master.lvclass">)
            n164 = call "0035H_浊度_第三点校正指令写入.vi"("数值"=u16 51, "MB session in"=w298) -> ("error out"=w299:errorcluster)  [unwired: 8 in, 1 out]
            n165 = case shown="错误" w299 {
              tunnel: [校准步骤."校准结果写入" ("元素") 校准步骤."放置第三点标液" ("元素")] -> w301
              frame No Error {
              }
              frame Error {
                n166 = global read "多参数全局变量.vi" "多参数编号"() -> (w308:string)
                n167 = Format Into String(format string="编号：%s\n参数：%s\n信息：%s" ("格式字符串"), w308, "浊度" ("输入 2"), "第三点校准异常，请重新校准！" ("error source (\" \")")) -> (resulting string=w307:string)  [unwired: 2 in, 1 out]
                n168 = One Button Dialog(message=w307) -> ()  [unwired: 1 in, 1 out]
              }
            }
            n169 = Enqueue Element(queue=w303, element=w301, timeout in ms (-1)=1000 ("超时毫秒(-1)")) -> ()  [unwired: 1 in, 3 out]
          }
        }
      }
      frame "第三点校准启动" {
        n170 = Greater Or Equal?(x=w314, y=60) -> (x >= y?=w320:bool)
        n171 = local read "最大值"() -> (w323:sgl)
        n172 = local read "最小值"() -> (w322:sgl)
        n173 = case shown="真" w320 {
          tunnel: [_ TRUE] -> w321
          frame False {
          }
          frame True {
          }
        }
        n174 = Subtract(x=w323, y=w322) -> (x-y=w324:sgl)
        n175 = Increment(x=w314) -> (x+1=w327:i32)
        n176 = Less Or Equal?(x=w324, y=10.0) -> (x <= y?=w317:bool)
        n177 = And(x=w317, y=w321) -> (x .and. y?=w325:bool)
        n178 = Greater Or Equal?(x=w327, y=180) -> (x >= y?=w326:bool)
        n179 = case shown="假" w325 {
          tunnel: w315 -> [w330 w342]
          tunnel: w326 -> [w331 _]
          tunnel: w327 -> [w329 _]
          tunnel: [w328 _] -> w312
          frame False {
            n180 = case shown="真" w331 {
              tunnel: w330 -> [_ w339]
              tunnel: w329 -> [w332 _]
              tunnel: [w332 _] -> w328
              frame False {
              }
              frame True {
                n181 = Enqueue Element(queue=w339, element=校准步骤."待机" ("元素")) -> ()  [unwired: 2 in, 3 out]
                n182 = global read "多参数全局变量.vi" "多参数编号"() -> (w336:string)
                n183 = Format Into String(format string="编号：%s\n参数：%s\n信息：%s" ("格式字符串"), w336, "浊度" ("输入 2"), "第三点校准超时，请重新校准！" ("error source (\" \")")) -> (resulting string=w334:string)  [unwired: 2 in, 1 out]
                n184 = One Button Dialog(message=w334) -> ()  [unwired: 1 in, 1 out]
              }
            }
          }
          frame True {
            n185 = Enqueue Element(queue=w342, element=校准步骤."第三点校准写入" ("元素"), timeout in ms (-1)=1000 ("超时毫秒(-1)")) -> ()  [unwired: 1 in, 3 out]
          }
        }
        n186 = Format Into String(format string="正在进行第三点校准,校准可能需要几分钟,请耐性等待,已进行%d秒." ("格式字符串"), w312) -> (resulting string=w313:string)  [unwired: 2 in, 1 out]
      }
      frame "第三点校准失败" {
      }
      frame "校准结果写入" {
        n187 = call "时间延迟"() -> ("error out"=w345:errorcluster)  [unwired: 11 in]
        n188 = local read "校准模式"() -> (w353:enum16{"两点校准", "单点校准", "三点校准"})
        n189 = Enqueue Element(queue=w354, element=校准步骤."校准结束" ("元素")) -> ()  [unwired: 2 in, 3 out]
        n190 = case shown="\"两点校准\", 默认" w353 {
          tunnel: [w358 w385] -> w348
          tunnel: w345 -> [_ _]
          frame "两点校准", Default {
            n191 = global read "国弘过程全局变量.vi" "Turb"() -> (w357:T3)
            n192 = Unbundle By Name(w357) -> ("电极状态标志"=w356:u16)
            n193 = case shown="33" w356 {
              selector: w356 -> [w360 _ _ w379]
              tunnel: [w359 w367 w375 w378] -> w358
              frame 0, Default {
                n194 = case shown="2, 32" w360 {
                  tunnel: ["校正未正常启动，请重新校正" "第一点校准通过" "第二点校准通过"] -> w359
                  frame 0, Default {
                  }
                  frame 1, 31 {
                  }
                  frame 2, 32 {
                  }
                }
              }
              frame 2 {
                n195 = local read "第一点校准值"() -> (w368:dbl)
                n196 = local read "第二点校准值"() -> (w365:dbl)
                n197 = local read "标液1"() -> (w369:dbl)
                n198 = local read "标液2"() -> (w364:dbl)
                n199 = Format Into String(format string="校准结果：第一点校准值=%f，第一点标准值=%f,第二点校准值=%f，第二点标准值=%f." ("提示"), w368, w369, w365, w364) -> (resulting string=w367:string)  [unwired: 2 in, 1 out]
              }
              frame 33 {
                n200 = local read "第一点校准值"() -> (w376:dbl)
                n201 = local read "第二点校准值"() -> (w374:dbl)
                n202 = local read "第三点校准值"() -> (w371:dbl)
                n203 = local read "标液1"() -> (w377:dbl)
                n204 = local read "标液2"() -> (w372:dbl)
                n205 = local read "标液3"() -> (w370:dbl)
                n206 = Format Into String(format string="校准结果：第一点校准值=%f，第一点标准值=%f,第二点校准值=%f，第二点标准值=%f,第三点校准值=%f，第三点标准值=%f." ("提示"), w376, w377, w374, w372, w371, w370) -> (resulting string=w375:string)  [unwired: 2 in, 1 out]
              }
              frame 3, 4 {
                n207 = case shown="3, 默认" w379 {
                  tunnel: ["校正失败，电极零点超出范围" "校正失败，电极斜率超出范围"] -> w378
                  frame 3, Default {
                  }
                  frame 4 {
                  }
                }
              }
            }
          }
          frame "单点校准" {
            n208 = local read "第一点校准值"() -> (w384:dbl)
            n209 = local read "标液1"() -> (w382:dbl)
            n210 = Format Into String(format string="校准结果：校准值=%f，标准值=%f。" ("提示"), w384, w382) -> (resulting string=w385:string)  [unwired: 2 in, 1 out]
          }
        }
        n211 = global read "多参数全局变量.vi" "多参数编号"() -> (w350:string)
        n212 = Format Into String(format string="编号：%s\n参数：%s\n信息：%s" ("格式字符串"), w350, "浊度" ("输入 2"), w348) -> (resulting string=w347:string)  [unwired: 2 in, 1 out]
        n213 = One Button Dialog(message=w347) -> ()  [unwired: 1 in, 1 out]
        n214 = call "操作日志.vi"("table"="校准记录", "日志信息"=w347) -> ("error out"=w352:errorcluster)  [unwired: 9 in]
      }
      frame "校准结束" {
        n215 = local read "提示"() -> (w386:string)
      }
    }
    "提示" <- w84
  }
